vi "Command Transmitter.vi"   [LabVIEW 2021]
uses:
  Type Definitions/Payload Class.ctl
  Type Definitions/Data Frame Header.ctl
  Type Definitions/Data Frame.ctl
  Type Definitions/Device.ctl
types:
  T1 = typedef "Data Frame.ctl" = cluster{"Frame Header":T2, "Payload":string, "CRC":u32}
  T2 = typedef "Data Frame Header.ctl" = cluster{"Sync":u32, "Time":dbl, "Nanosecond Counter":i64, "Payload Class":T3, "Payload ID":u16, "Counter":i32, "Options":u32, "Source":T4, "Destination":T4}
  T3 = typedef "Payload Class.ctl" = enum16{"System State", "Parameters", "Metadata", "Software Monitor", "Data", "Commands"}
  T4 = typedef "Device.ctl" = enum32{"None", "Exec", "Aux1", "Aux2", "Aux3"}
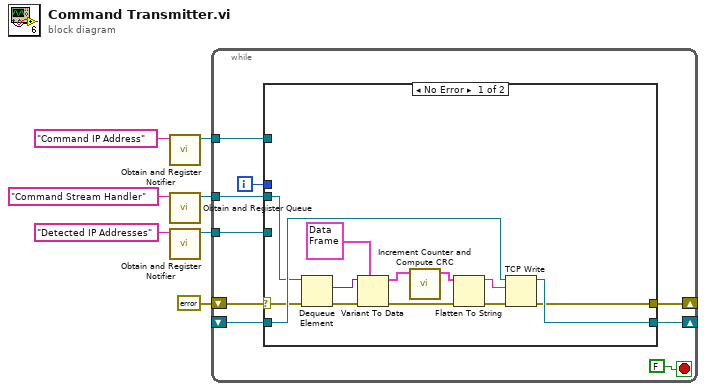
[diagram p0: block diagram]
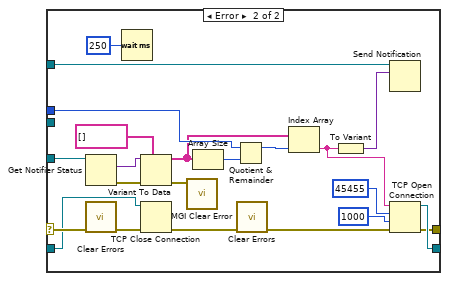
[diagram p2: hidden frame]
diagram:
  n1 = call "Obtain and Register Notifier.vi"("name (unnamed)"="Command IP Address") -> ("notifier out"=w7:refnum<notifier>)  [unwired: 8 in, 2 out]
  n2 = call "Obtain and Register Queue.vi"("name (unnamed)"="Command Stream Handler") -> ("Queue Out"=w2:refnum<queue>)  [unwired: 7 in, 3 out]
  n3 = call "Obtain and Register Notifier.vi"("name (unnamed)"="Detected IP Addresses") -> ("notifier out"=w5:refnum<notifier>)  [unwired: 8 in, 2 out]
  n4 = while {
    shift-right: [w16] -> _
    shift-left: errorcluster {"status"=TRUE, "code"=0, "source"=""} ("error out") -> [w11]
    shift-right: [w15] -> _
    shift-left: _ -> [w14]
    tunnel: w2 -> [w12]
    tunnel: w5 -> [w9]
    tunnel: w7 -> [w8]
    i -> [w10]
    stop <- FALSE stop-if-true
    n5 = case shown="No Error" w11 {
      selector: w11 -> [w17 w51]
      tunnel: [w27 w44] -> w16
      tunnel: [w28 w46] -> w15
      tunnel: w14 -> [w29 w47]
      tunnel: w12 -> [w26 _]
      tunnel: w10 -> [_ w39]
      tunnel: w9 -> [_ w38]
      tunnel: w8 -> [_ w32]
      frame No Error {
        n6 = Dequeue Element(queue=w26, error in (no error)=w17) -> (element=w23:variant, error out=w18:errorcluster)  [unwired: 1 in, 2 out]
        n7 = Variant To Data(error in=w18, type=T1 {"Frame Header"={"Sync"=0, "Time"=0.0, "Nanosecond Counter"=0, "Payload Class"=enum."System State", "Payload ID"=0, "Counter"=0, "Options"=0, "Source"=enum."None", "Destination"=enum."None"}, "Payload"="", "CRC"=0} ("Frame"), Variant=w23) -> (data=w22:T1, error out=w19:errorcluster)
        n8 = call "Increment Counter and Compute CRC.vi"("Frame In"=w22) -> ("Frame Out"=w21:T1)  [unwired: 9 in, 1 out]
        n9 = Flatten To String(anything=w21, error in (no error)=w19) -> (data string=w24:string, error out=w20:errorcluster)  [unwired: 2 in, 1 out]
        n10 = TCP Write(connection ID=w29, data in=w24, error in (no error)=w20) -> (connection ID out=w28:refnum<k5>, error out=w27:errorcluster)  [unwired: 1 in, 1 out]
      }
      frame Error {
        n11 = Get Notifier Status(notifier=w38) -> (current notification=w37:variant, error out=w34:errorcluster)  [unwired: 1 in, 3 out]
        n12 = call <vilib>:"Clear Errors.vi"("error in (no error)"=w51) -> ("error out"=w49:errorcluster)  [unwired: 5 in, 1 out]
        n13 = Wait (ms)(milliseconds to wait=u32 250) -> ()  [unwired: 1 out]
        n14 = Variant To Data(error in=w34, type=string[] [] ("Adapter IP Addresses"), Variant=w37) -> (data=w35:string[], error out=w33:errorcluster)
        n15 = TCP Close Connection(connection ID=w47, error in (no error)=w49) -> (error out=w48:errorcluster)  [unwired: 1 in, 1 out]
        n16 = call <userlib>:"MGI Clear Error.vi"("Error In"=w33) -> ()  [unwired: 6 in, 1 out]
        n17 = Array Size(array=w35) -> (size(s)=w40:i32)
        n18 = Quotient & Remainder(x=w39, y=w40) -> (x-y*floor(x/y)=w41:i32)  [unwired: 1 out]
        n19 = call <vilib>:"Clear Errors.vi"("error in (no error)"=w48) -> ("error out"=w45:errorcluster)  [unwired: 5 in, 1 out]
        n20 = Index Array(array=w35, index=w41) -> (element=w31:string)
        n21 = To Variant(anything=w31) -> (Variant=w30:variant)
        n22 = Send Notification(notification=w30, notifier=w32) -> ()  [unwired: 1 in, 2 out]
        n23 = TCP Open Connection(address=w31, remote port or service name=u16 45455 ("port"), timeout ms (60000)=1000 ("timeout ms (wait forever: -1)"), error in (no error)=w45) -> (connection ID=w46:refnum<k5>, error out=w44:errorcluster)  [unwired: 1 in]
      }
    }
  }
